vi "FPGA_Main.vi"() -> ()   [LabVIEW 2016]
uses:
  <vilib>/Platform/TimedLoop/XDataNode/timing_clust.ctl
  <vilib>/Platform/TimedLoop/XDataNode/nitl_modes.ctl
  <vilib>/Platform/TimedLoop/XDataNode/wakeup.ctl
  <vilib>/rvi/FXPMathLib/FxpSinAndCos/subVIs/nifxpmath_SinAndCos_SimConfig.ctl
  <vilib>/rvi/FXPMathLib/FxpConvert/subVIs/nifxpmath_Convert_SimConfig.ctl
  <vilib>/fxp/LVFixedPointQuantizationPolicyTypeDef.ctl
  <vilib>/fxp/LVFixedPointOverflowPolicyTypeDef.ctl
  <vilib>/rvi/FXPMathLib/basic elements/DSP48E/simVIs/niFpgaDsp48eSimulationState.ctl
  <vilib>/rvi/FXPMathLib/basic elements/DSP48E/subVIs/niFpgaDsp48eType.ctl
  <vilib>/rvi/FXPMathLib/basic elements/DSP48E/subVIs/niFpgaDsp48eAlumodeOpmodeCarryinselState.ctl
  <vilib>/rvi/FXPMathLib/basic elements/DSP48E/subVIs/niFpgaDsp48eUseMultiplierState.ctl
  <vilib>/rvi/FXPMathLib/basic elements/DSP48E/subVIs/niFpgaDsp48eLogicUnitModeState.ctl
  <vilib>/rvi/FXPMathLib/basic elements/DSP48E/subVIs/niFpgaDsp48eSelectPatternState.ctl
  <vilib>/rvi/FXPMathLib/basic elements/DSP48E/subVIs/niFpgaDsp48eSelectMaskState.ctl
  <vilib>/rvi/FXPMathLib/basic elements/DSP48E/subVIs/niFpgaDsp48eAutoresetState.ctl
  <vilib>/rvi/FXPMathLib/basic elements/DSP48E/subVIs/niFpgaDsp48eSimulationConfig.ctl
  <vilib>/rvi/FXPMathLib/basic elements/DSP48E/simVIs/niFpgaDsp48eResets.ctl
  <vilib>/rvi/FXPMathLib/basic elements/DSP48E/simVIs/niFpgaDsp48eEnables.ctl
  <vilib>/rvi/FXPMathLib/basic elements/DSP48E/simVIs/niFpgaDsp48eRegisters.ctl
  <vilib>/rvi/Emulation/niFpgaGetClockAttributes.vi
  <vilib>/rvi/Emulation/niFpgaSctlEmulationGetInTimedLoop.vi
  <vilib>/rvi/Emulation/niFpgaEmulationReportErrorSimple.vi
  <vilib>/rvi/Emulation/niFpgaEmulationIsFPGAContextNoSignature.vi
  <vilib>/rvi/FIFO/Fifo_Resource/nirvififoEmulationSetSize.vi
  <vilib>/rvi/DataTransferAndStorage/Container/Common/niFpgaContainerGetUniqueNameForEmu.vi
  <vilib>/rvi/FIFO/Fifo_Resource/nirviFifoEmulationQueueMgr.vi
  <instcachedir>/0/nirviFifoEmulationQueueMgr_E5CAEC123FF24DC58D834DCA3CDAA9B5.lvgen/nirviFifoEmulationQueueMgr_E5CAEC123FF24DC58D834DCA3CDAA9B5_012.vi
  <vilib>/rvi/Emulation/niFpgaProcessEmulError.vi
  <vilib>/rvi/Emulation/niFpgaCriticalErrorInLSC.vi
  <vilib>/rvi/errors/niFpgaSetErrorForExecOnDevCompSimple.vi
  <vilib>/rvi/eio/common/nirviEmuReportErrorAndStop.vi
  <vilib>/rvi/FIFO/Fifo_Resource/nirvififoEmulationDetermineInputValidOut.vi
  <vilib>/rvi/FIFO/Fifo_Resource/nirvififoEmulationCreateLock.vi
  <vilib>/rvi/FIFO/Fifo_Resource/nirvififoEmulationObtainLock.vi
  <vilib>/rvi/FIFO/Fifo_Resource/nirvififoEmulationReleaseLock.vi
  <vilib>/rvi/occurrence/nirviWaitOnOccurrenceBase.vi
  <vilib>/rvi/errors/nirviReportUnexpectedCaseInternalError.vi
  <vilib>/rvi/errors/nirviReportUnexpectedCaseInternalError (U32).vi
  <vilib>/rvi/FXPMathLib/FxpSinAndCos/simVIs/DllFxpSinAndCosTemp_sub.vi
  <vilib>/rvi/FXPMathLib/FxpConvert/simVIs/DllFxpConvertTemp_sub.vi
  <vilib>/Utility/error.llb/Clear Errors.vi
  <vilib>/rvi/FXPMathLib/basic elements/DSP48E/subVIs/niFpgaDsp48eCheckOwningTarget.vi
  <vilib>/rvi/FXPMathLib/basic elements/DSP48E/subVIs/niFpgaDsp48eCheckIfOnUltraScale.vi
  <vilib>/rvi/FXPMathLib/basic elements/DSP48E/simVIs/niFpgaDsp48eCheckMode.vi
  <vilib>/rvi/FXPMathLib/basic elements/DSP48E/simVIs/niFpgaDsp48eReportInvalidMode.vi
  <vilib>/rvi/FXPMathLib/basic elements/DSP48E/simVIs/niFpgaDsp48eSimMultiplier.vi
  <vilib>/rvi/FXPMathLib/basic elements/DSP48E/simVIs/niFpgaDsp48eSimArithmetic.vi
  <vilib>/rvi/FXPMathLib/basic elements/DSP48E/simVIs/niFpgaDsp48eSimPatternDetect.vi
  <vilib>/rvi/FXPMathLib/basic elements/DSP48E/simVIs/niFpgaDsp48eSimP.vi
  <vilib>/rvi/FXPMathLib/basic elements/DSP48E/simVIs/niFpgaDsp48eSimUpdateState.vi
  <vilib>/rvi/interface/RandomDataEmulation/niFpgaRandomDataHandleErrors.vi
  <vilib>/rvi/DataTransferAndStorage/Container/XNode/niFpgaContainer.xnode
  <vilib>/rvi/FIFO/Fifo_Resource/nirvififoEmulationClear.vi
  <vilib>/Platform/TimedLoop/XDataNode/XDataNode.xnode
  <vilib>/rvi/FIFO/Fifo_Resource/nirvififoEmulationWrite.vi
  <vilib>/rvi/FXPMathLib/FxpAdd/XNode/nifxpmath_Add.xnode
  <vilib>/rvi/FXPMathLib/FxpSinAndCos/XNode/nifxpmath_SinAndCos.xnode
  <vilib>/rvi/FXPMathLib/FxpConvert/XNode/nifxpmath_Convert.xnode
  <vilib>/rvi/FIFO/Fifo_Resource/nirvififoEmulationRead.vi
  <vilib>/rvi/FXPMathLib/basic elements/DSP48E/XNode/niFpgaDsp48e.xnode
  <vilib>/rvi/interface/RandomDataEmulation/nirviRandomDataFpgaReadWriteTemplate.vi
  <vilib>/Platform/TimedLoop/XDataNode/XDNodeRunTimeDep.lvlib
  <vilib>/rvi/FXPMathLib/sim/FxpSim.dll
panel:
  in  "aReset":bool
  in  "Phase Increment":fxp<+/-,16,1>
  in  "LPF Enable":bool
  in  "AWGN Enable":bool
  in  "RMS Noise":u16=1024
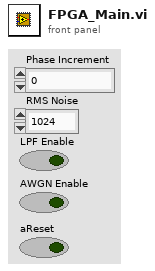
[diagram p1: front panel]
types:
  T1 = typedef "XDNodeRunTimeDep.lvlib/timing_clust.ctl" = cluster{"Expected End [f-1]":u64, "Actual End [f-1]":u64, "Finished Late? [f-1]":bool, "Expected End [i-1]":u64, "Actual End [i-1]":u64, "Finished Late? [i-1]":bool, "Expected Start [i]":u64, "Actual Start [i]":u64, "Expected Start [f]":u64, "Actual Start [f]":u64, "Source Name":string, "Structure Name":string, "Period":i64, "Deadline":i64, "Offset":i64, "Start":i64, "Priority":i32, "Timeout":i32, "Mode":T2, "Wakeup Reason":T3, "Error":errorcluster, "Source Type":string, "Secondary Source Type":string, "Global End Time":u64, "Global Start Time":u64, "Frame Duration":u64, "Iteration Duration":u64, "Assigned CPU":i32, "I/O Scan Engine Mode":u32}
  T2 = typedef "XDNodeRunTimeDep.lvlib/nitl_modes.ctl" = enum32{"No Change", "Process missed periods, maintain original phase", "Discard missed periods, maintain original phase", "Process missed periods, ignore original phase", "Discard missed periods, ignore original phase"}
  T3 = typedef "XDNodeRunTimeDep.lvlib/wakeup.ctl" = enum32{"Normal", "Aborted", "Asynchronous wakeup", "Timing source error", "Timed loop error", "Timeout"}
  T4 = typedef "niFpgaDsp48eRegisters.ctl" = cluster{"a register 1":fxp<+/-,30,30>, "a register 2":fxp<+/-,30,30>, "b register 1":fxp<+/-,18,18>, "b register 2":fxp<+/-,18,18>, "c register":fxp<+/-,48,48>, "d register":fxp<+/-,25,25>, "ad register":fxp<+/-,27,27>, "m register":fxp<+/-,45,45>, "opmode register":fxp<+,7,7>, "alumode register":fxp<+,4,4>, "carryinsel register":fxp<+,3,3>, "inmode register":fxp<+,5,5>, "carryin register":bool, "multcarryin register":bool, "p registers":fxp<+/-,48,48>, "carryout register":fxp<+,4,4>, "carrycascout register":bool, "multsignout register":bool, "patterndetect register":bool, "patternbdetect register":bool, "patterndetect register 2":bool, "patternbdetect register 2":bool}
  T5 = typedef "niFpgaDsp48eEnables.ctl" = cluster{"cea1":bool, "cea2":bool, "cead":bool, "cealumode":bool, "ceb1":bool, "ceb2":bool, "cec":bool, "cecarryin":bool, "cectrl":bool, "ced":bool, "ceinmode":bool, "cem":bool, "cemultcarryin":bool, "cep":bool}
  T6 = typedef "niFpgaDsp48eResets.ctl" = cluster{"rsta":bool, "rstallcarryin":bool, "rstalumode":bool, "rstb":bool, "rstc":bool, "rstctrl":bool, "rstd":bool, "rstinmode":bool, "rstm":bool, "rstp":bool}
  T7 = typedef "niFpgaDsp48eSimulationConfig.ctl" = enum16{"Use 25x18", "Use 27x18"}
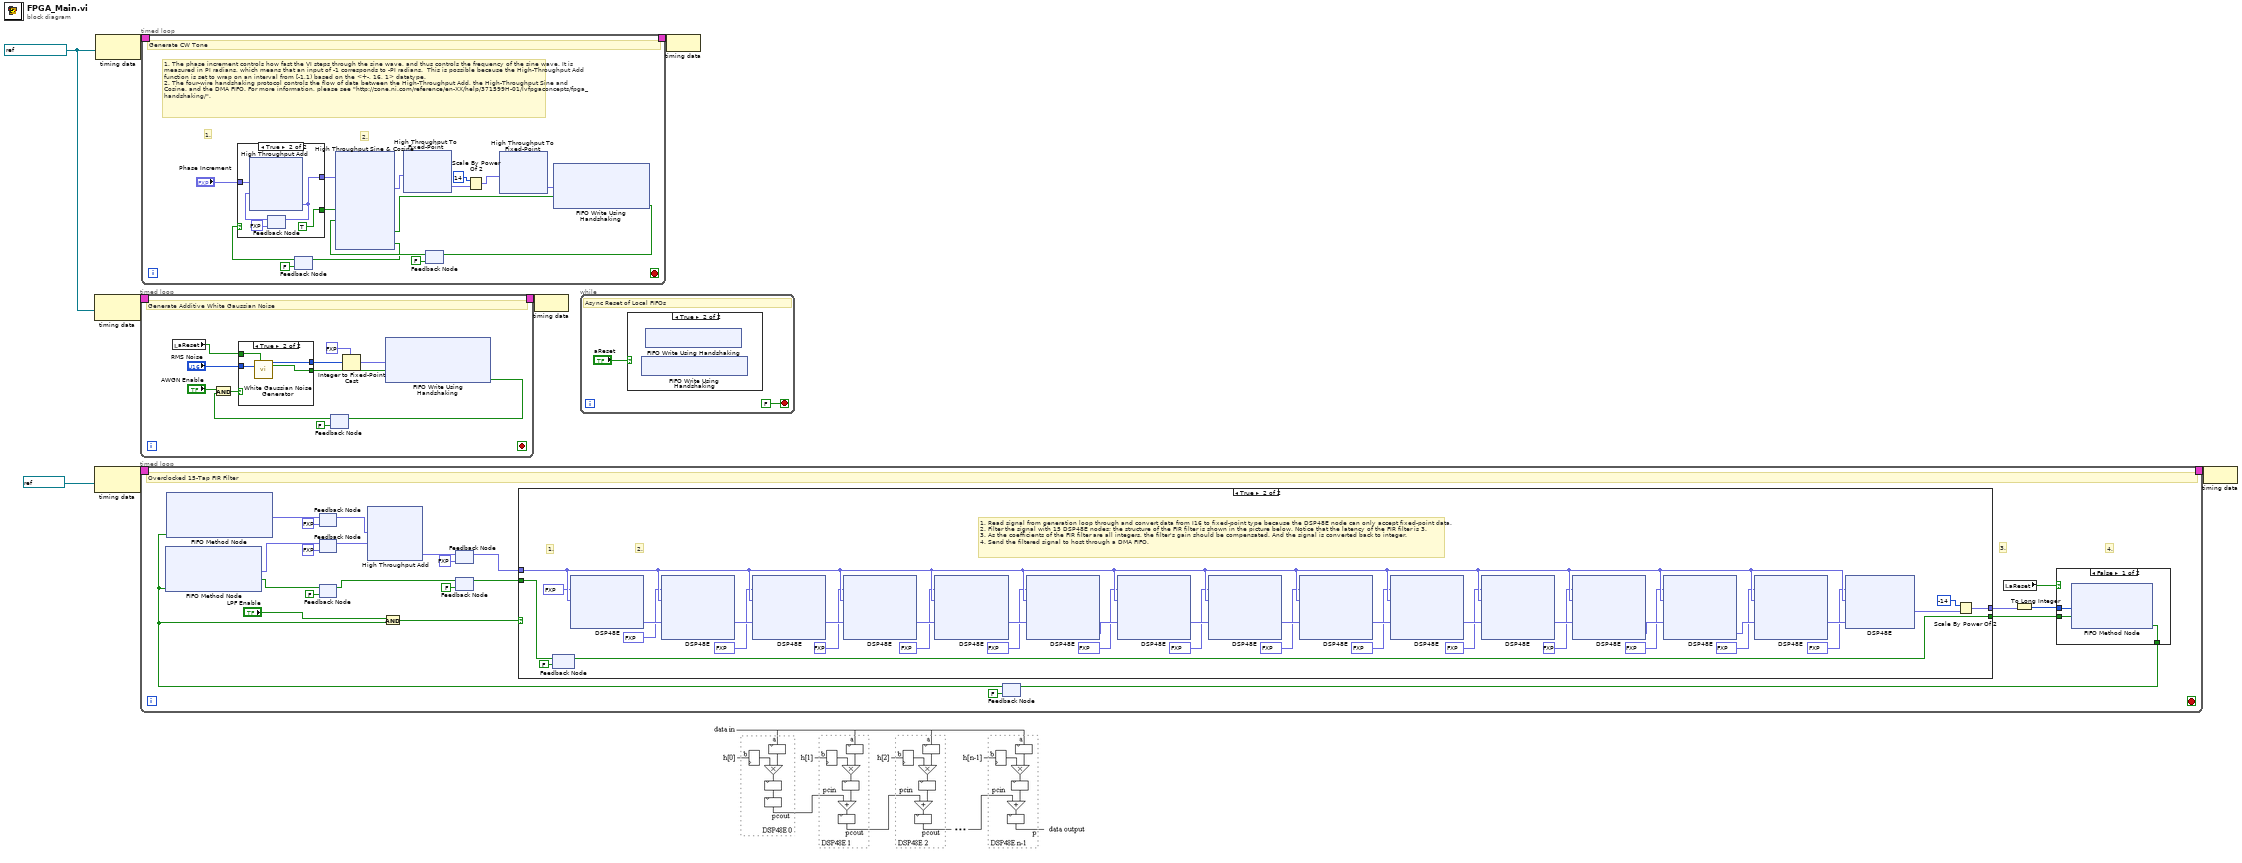
[diagram p0: block diagram]
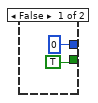
[diagram p3: hidden frame]
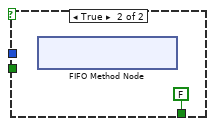
[diagram p4: hidden frame]
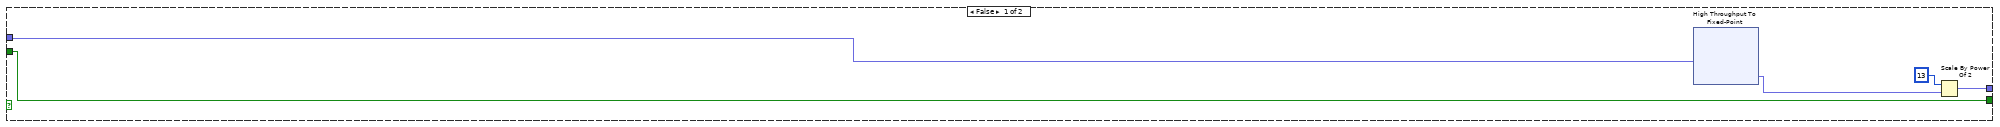
[diagram p5: hidden frame]
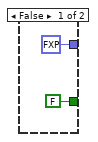
[diagram p6: hidden frame]
diagram:
  w2 = refnum<k21> "100 MHz Clock" ("Source Name")
  n1 = node-c288(w2) -> (w4:T1)
  n2 = node-c288(refnum<k21> "160MHz" ("Source Name")) -> (w6:T1)
  n3 = node-c288(w2) -> (w8:T1)
  n4 = timed-loop {
    timing: w4 -> [_]
    timing-out: [_] -> w3
    stop <- _ stop-if-true
    # "Generate Additive White Gaussian Noise"
    n5 = local read "aReset"() -> (w12:bool)
    n6 = feedback #1(FALSE ("Ready for Input")) -> (w14:bool)
    n7 = And(x="AWGN Enable", y=w14) -> (x .and. y?=w17:bool)
    n8 = case shown="True" w17 {
      tunnel: "RMS Noise" -> [_ w25]
      tunnel: [i16 0 ("white noise out") w24] -> w11
      tunnel: [TRUE ("data valid?") w23] -> w18
      tunnel: w12 -> [_ w22]
      frame False {
      }
      frame True {
        n9 = call "White Gaussian Noise Generator"("reset"=w22, "RMS"=w25) -> ("white noise out"=w24:i16, "data valid?"=w23:bool)  [unwired: 12 in]
      }
    }
    n10 = Integer to Fixed-Point Cast(fixed-point type=fxp<+/-,17,17> 0.0, integer=w11) -> (fixed-point=w10:fxp<+/-,17,17>)
    n11 = xnode ("FIFO Write Using Handshaking")("Element"=w10, "Input Valid"=w18) -> ("Ready for Input"=w15:bool)  [unwired: 1 in, 1 out]
    n12 = feedback-in #1(w15) -> ()
  }
  n13 = timed-loop {
    timing: w6 -> [_]
    timing-out: [_] -> w5
    stop <- _ stop-if-true
    # "3."
    # "4."
    # "Overclocked 15-Tap FIR Filter"
    n14 = feedback #2(fxp<+/-,17,17> 0.0 ("Element")) -> (w37:fxp<+/-,17,17>)
    n15 = feedback #3(fxp<+/-,17,17> 0.0 ("Element")) -> (w36:fxp<+/-,17,17>)
    n16 = feedback #4(FALSE ("Output Valid")) -> (w28:bool)
    n17 = xnode ("High Throughput Add")("x"=w37, "y"=w36) -> ("x+y"=w43:fxp<+/-,18,18>)
    n18 = feedback-in #5(w43) -> ()
    n19 = feedback #5(fxp<+/-,18,18> 0.0 ("x+y")) -> (w33:fxp<+/-,18,18>)
    n20 = feedback-in #6(w28) -> ()
    n21 = feedback #6(FALSE) -> (w32:bool)
    n22 = feedback #7(FALSE ("Ready for Input")) -> (w44:bool)
    n23 = xnode ("FIFO Method Node")("Ready for Output"=w44) -> ("Element"=w38:fxp<+/-,17,17>, "Output Valid"=w50:bool)  [unwired: 1 in, 1 out]
    n24 = xnode ("FIFO Method Node")("Ready for Output"=w44) -> ("Element"=w39:fxp<+/-,17,17>)  [unwired: 1 in, 2 out]
    n25 = feedback-in #2(w39) -> ()
    n26 = feedback-in #3(w38) -> ()
    n27 = feedback-in #4(w50) -> ()
    n28 = And(x="LPF Enable", y=w44) -> (x .and. y?=w45:bool)
    n29 = case shown="True" w45 {
      tunnel: w33 -> [w56 w117]
      tunnel: [w57 w83] -> w29
      tunnel: w32 -> [w59 w86]
      tunnel: [w59 w85] -> w49
      frame False {
        n30 = xnode ("High Throughput To Fixed-Point")("x"=w56) -> ("y"=w55:fxp<+/-,33,33>)
        n31 = Scale By Power Of 2(n=i16 13, x=w55) -> (x*2^n=w57:fxp<+/-,33,33>)
      }
      frame True {
        # "1. Read signal from generation loop through and convert data from I16 to fixed-point type because the DSP48E node can only accept fixed-point data.\n2. Filter the signal with 15 DSP48E nodes; the structure of the FIR filter is shown in the picture below. Notice that the latency of the FIR filter is 3.\n3. As the coefficients of the FIR filter are all integers, the filter's gain should be compensated. And the signal is converted back to integer.\n4. Send the filtered signal to host through a DMA FIFO."
        # "2."
        # "1."
        n32 = feedback #8(FALSE ("Timed Out?")) -> (w85:bool)
        n33 = feedback-in #8(w86) -> ()
        n34 = xnode ("DSP48E")("a"=fxp<+/-,30,30> -4125.0, "b"=w117) -> ("pcout"=w115:fxp<+/-,48,48>)  [unwired: 1 out]
        n35 = xnode ("DSP48E")("a"=fxp<+/-,30,30> -6954.0, "b"=w117, "pcin"=w115) -> ("pcout"=w113:fxp<+/-,48,48>)  [unwired: 1 out]
        n36 = xnode ("DSP48E")("a"=fxp<+/-,30,30> -5900.0, "b"=w117, "pcin"=w113) -> ("pcout"=w111:fxp<+/-,48,48>)  [unwired: 1 out]
        n37 = xnode ("DSP48E")("a"=fxp<+/-,30,30> 0.0, "b"=w117, "pcin"=w111) -> ("pcout"=w109:fxp<+/-,48,48>)  [unwired: 1 out]
        n38 = xnode ("DSP48E")("a"=fxp<+/-,30,30> 9834.0, "b"=w117, "pcin"=w109) -> ("pcout"=w108:fxp<+/-,48,48>)  [unwired: 1 out]
        n39 = xnode ("DSP48E")("a"=fxp<+/-,30,30> 20861.0, "b"=w117, "pcin"=w108) -> ("pcout"=w107:fxp<+/-,48,48>)  [unwired: 1 out]
        n40 = xnode ("DSP48E")("a"=fxp<+/-,30,30> 29502.0, "b"=w117, "pcin"=w107) -> ("pcout"=w106:fxp<+/-,48,48>)  [unwired: 1 out]
        n41 = xnode ("DSP48E")("a"=fxp<+/-,30,30> 32767.0, "b"=w117, "pcin"=w106) -> ("pcout"=w105:fxp<+/-,48,48>)  [unwired: 1 out]
        n42 = xnode ("DSP48E")("a"=fxp<+/-,30,30> 29502.0, "b"=w117, "pcin"=w105) -> ("pcout"=w104:fxp<+/-,48,48>)  [unwired: 1 out]
        n43 = xnode ("DSP48E")("a"=fxp<+/-,30,30> 20861.0, "b"=w117, "pcin"=w104) -> ("pcout"=w103:fxp<+/-,48,48>)  [unwired: 1 out]
        n44 = xnode ("DSP48E")("a"=fxp<+/-,30,30> 9834.0, "b"=w117, "pcin"=w103) -> ("pcout"=w102:fxp<+/-,48,48>)  [unwired: 1 out]
        n45 = xnode ("DSP48E")("a"=fxp<+/-,30,30> 0.0, "b"=w117, "pcin"=w102) -> ("pcout"=w101:fxp<+/-,48,48>)  [unwired: 1 out]
        n46 = xnode ("DSP48E")("a"=fxp<+/-,30,30> -5900.0, "b"=w117, "pcin"=w101) -> ("pcout"=w100:fxp<+/-,48,48>)  [unwired: 1 out]
        n47 = xnode ("DSP48E")("a"=fxp<+/-,30,30> -6954.0, "b"=w117, "pcin"=w100) -> ("pcout"=w99:fxp<+/-,48,48>)  [unwired: 1 out]
        n48 = xnode ("DSP48E")("a"=fxp<+/-,30,30> -4125.0, "b"=w117, "pcin"=w99) -> ("p"=w84:fxp<+/-,48,48>)
        n49 = Scale By Power Of 2(n=i16 -14, x=w84) -> (x*2^n=w83:fxp<+/-,48,48>)
      }
    }
    n50 = local read "aReset"() -> (w42:bool)
    n51 = To Long Integer(number=w29) -> (32bit integer=w41:i32)
    n52 = case shown="False" w42 {
      tunnel: w41 -> [w53 _]
      tunnel: w49 -> [w52 _]
      tunnel: [w51 FALSE ("Ready for Input")] -> w48
      frame False {
        n53 = xnode ("FIFO Method Node")("Element"=w53, "Input Valid"=w52) -> ("Ready for Input"=w51:bool)  [unwired: 1 in, 1 out]
      }
      frame True {
        n54 = xnode ("FIFO Method Node")() -> ()  [unwired: 1 in, 1 out]
      }
    }
    n55 = feedback-in #7(w48) -> ()
  }
  n56 = timed-loop {
    timing: w8 -> [_]
    timing-out: [_] -> w7
    stop <- _ stop-if-true
    # "1. The phase increment controls how fast the VI steps through the sine wave, and thus controls the frequency of the sine wave. It is measured in PI radians, which means that an input of -1 corresponds to -PI radians.  This is possible because the High-Throughput Add function is set to wrap on an interval from [-1,1) based on the <+-, 16, 1> datatype.\n2. The four-wire handshaking protocol controls the flow of data between the High-Throughput Add, the High-Throughput Sine and Cosine. and the DMA FIFO. For more information, please see \"http://zone.ni.com/reference/en-XX/help/371599H-01/lvfpgaconcepts/fpga_handshaking/\"."
    # "1."
    # "2."
    # "Generate CW Tone"
    n57 = feedback #9(FALSE ("ready for input")) -> (w1392:bool)
    n58 = case shown="True" w1392 {
      tunnel: "Phase Increment" -> [_ w1443]
      tunnel: [fxp<+/-,16,1> 0.0 ("x+y") w1442] -> w1386
      tunnel: [FALSE TRUE] -> w1393
      frame False {
      }
      frame True {
        n59 = feedback #10(fxp<+/-,16,1> 0.0 ("x+y")) -> (w1445:fxp<+/-,16,1>)
        n60 = xnode ("High Throughput Add")("x"=w1443, "y"=w1445) -> ("x+y"=w1442:fxp<+/-,16,1>)
        n61 = feedback-in #10(w1442) -> ()
      }
    }
    n62 = feedback #11(FALSE ("Ready for Input")) -> (w1394:bool)
    n63 = xnode "High Throughput Sine & Cosine"("x (pi)"=w1386, "input valid"=w1393, "ready for output (T)"=w1394) -> ("sin(x)"=w1385:fxp<+/-,16,2>, "output valid"=w1387:bool, "ready for input"=w1390:bool)  [unwired: 1 out]
    n64 = feedback-in #9(w1390) -> ()
    n65 = xnode "High Throughput To Fixed-Point"("x"=w1385) -> ("y"=w1384:fxp<+/-,31,17>)
    n66 = Scale By Power Of 2(n=i16 14, x=w1384) -> (x*2^n=w1381:fxp<+/-,31,17>)
    n67 = xnode "High Throughput To Fixed-Point"("x"=w1381) -> ("y"=w1382:fxp<+/-,17,17>)
    n68 = xnode ("FIFO Write Using Handshaking")("Element"=w1382, "Input Valid"=w1387) -> ("Ready for Input"=w1389:bool)  [unwired: 1 in, 1 out]
    n69 = feedback-in #11(w1389) -> ()
  }
  n70 = node-c288(w3) -> ()
  n71 = while {
    stop <- FALSE stop-if-true
    # "Async Reset of Local FIFOs"
    n72 = case shown="True" "aReset" {
      frame False {
      }
      frame True {
        n73 = xnode ("FIFO Write Using Handshaking")() -> ()  [unwired: 1 in, 1 out]
        n74 = xnode ("FIFO Write Using Handshaking")() -> ()  [unwired: 1 in, 1 out]
      }
    }
  }
  n75 = node-c288(w7) -> ()
  n76 = node-c288(w5) -> ()
